vi "_UtilsRandomDBLArray.vi"(1 "array size":i32=256, 2 "factor":dbl=1.0) -> (0 "array":dbl[](array[numeric]))   [LabVIEW 2014, in "examples.lvlib"]
uses:
  examples.lvlib
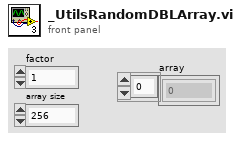
[diagram p1: front panel]
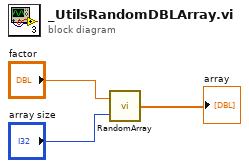
[diagram p0: block diagram]
diagram:
  n1 = call "RandomArray.vi"("random array size"="array size", "factor"="factor") -> ("random array"=→"array":dbl[])
